vi "GEOM_All2LLcoords.vi"(9 "Amplifiers":T1[](array[typedef]) {"fliped" items=["none", "horizontal", "vertical"]; "type" items=["LL", "LR", "UL", "UR"]}) -> (1 "Amps with LL ROIs":T1[](array[typedef]) {"fliped" items=["none", "horizontal", "vertical"]; "type" items=["LL", "LR", "UL", "UR"]})   [LabVIEW 2016]
uses:
  GEOM_Amplifier.ctl
  GEOM_AmpType.ctl
  GEOM_ROI.ctl
  GEOM_Coords.ctl
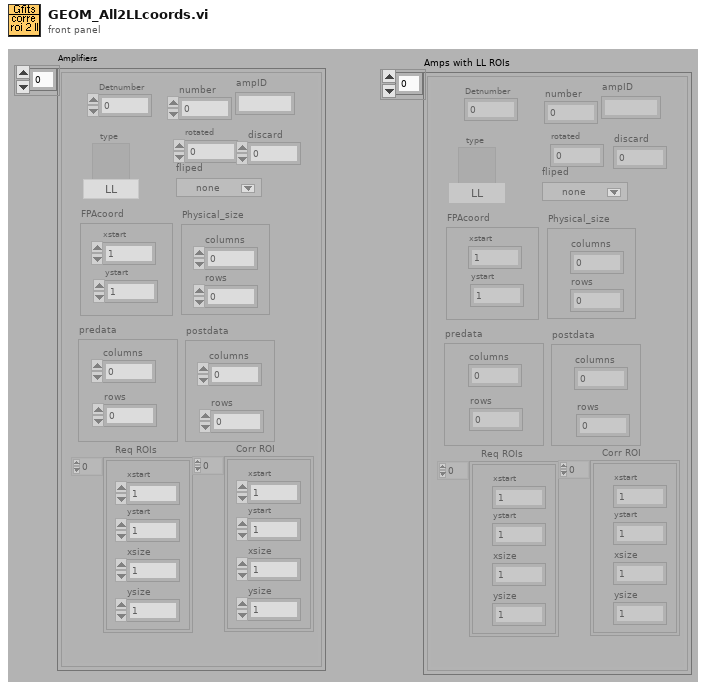
[diagram p1: front panel]
types:
  T1 = typedef "GEOM_Amplifier.ctl" = cluster{"number":i32, "type":T2, "rotated":i16, "fliped":u16, "FPAcoord":cluster{"xstart":i32, "ystart":i32}, "Physical_size":cluster{"columns":i32, "rows":i32}, "predata":cluster{"columns":i32, "rows":i32}, "postdata":cluster{"columns":i32, "rows":i32}, "Req ROIs":T3, "Corr ROI":T3, "Detnumber":i32, "ampID":string, "discard":i32}
  T2 = typedef "GEOM_AmpType.ctl" = u16
  T3 = typedef "GEOM_ROI.ctl" = T4[]
  T4 = typedef "GEOM_Coords.ctl" = cluster{"xstart":u32, "ystart":u32, "xsize":u32, "ysize":u32}
  T5 = cluster{"xstart":i32, "ystart":i32, "xend":i32, "yend":i32}
  T6 = cluster{"xstart":i32, "ystart":i32, "xsize":i32, "ysize":i32}
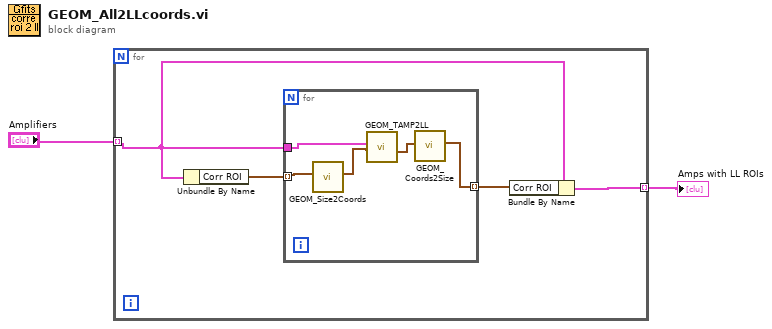
[diagram p0: block diagram]
diagram:
  n1 = for {
    tunnel: "Amplifiers" -> [w5] mode=indexing
    tunnel: [w3] -> w1 mode=indexing
    n2 = Unbundle By Name(w5) -> ("Corr ROI"=w6:T3)
    n3 = for {
      tunnel: w5 -> [w8]
      tunnel: w6 -> [w11] mode=indexing
      tunnel: [w7] -> w4 mode=indexing
      n4 = call "GEOM_Size2Coords.vi"("Size"=w11) -> ("Coords"=w10:T5)  [unwired: 10 out]
      n5 = call "GEOM_TAMP2LL.vi"("AMPROIcoords"=w10, "Amplifier"=w8) -> ("DETROICoords"=w9:T5)  [unwired: 9 out]
      n6 = call "GEOM_Coords2Size.vi"("Coords"=w9) -> ("Size"=w7:T6)  [unwired: 10 out]
    }
    n7 = Bundle By Name(cluster=w5, "Corr ROI"=w4) -> (w3:T1)
  }
  "Amps with LL ROIs" <- w1
